vi "Set Dev Bounds.vi"(7 "error in (no error)":errorcluster, 8 "firmware revision":string(combo), 9 "dev bounds":T2={"dev bound upper cap (101)"=101.0, "dev bound upper loss (0.1)"=0.1, "dev bound lower cap (99)"=99.0, "dev bound lower loss (-0.1)"=-0.1}, 10 "VISA resource name":refnum<visa-resource-name>) -> (0 "error out":errorcluster, 2 "bridge error":T1, 3 "VISA resource name out":refnum<visa-resource-name>)   [LabVIEW 2019, in "Andeen-Hagerling 2700A.lvlib"]
doc: "Set the value of the value of the deviation mode bounds parameters.\n\nThis is the upper and lower bounds of the deviation capacitance\nand loss spans in pF and jpF respectively. The capacitance\nand loss bounds correspond directly to the analog output\nvoltage bounds for capacitance and loss respectively."
uses:
  Andeen-Hagerling 2700A.lvlib
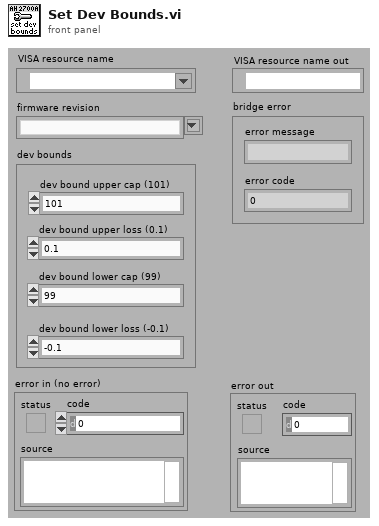
[diagram p1: front panel]
types:
  T1 = cluster{"error message":string, "error code":i32}
  T2 = cluster{"dev bound upper cap (101)":dbl, "dev bound upper loss (0.1)":dbl, "dev bound lower cap (99)":dbl, "dev bound lower loss (-0.1)":dbl}
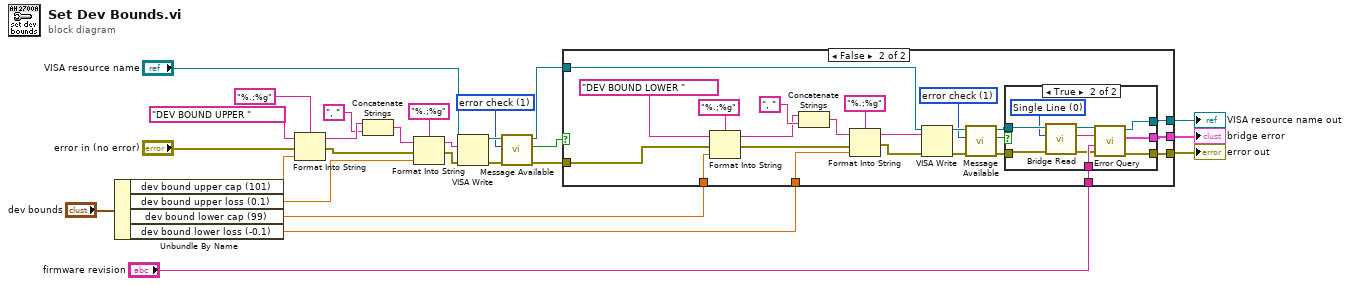
[diagram p0: block diagram]
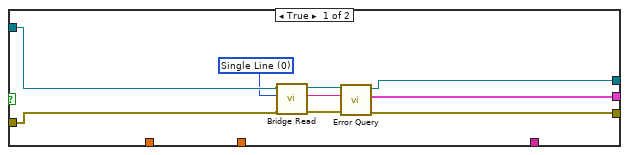
[diagram p2: hidden frame]
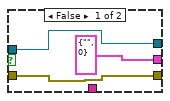
[diagram p3: hidden frame]
diagram:
  w1 = u16 1 items=["none", "error check", "multiline read", "infinite"] ("delay")
  n1 = Unbundle By Name("dev bounds") -> ("dev bound upper cap (101)"=w17:dbl, "dev bound upper loss (0.1)"=w16:dbl, "dev bound lower cap (99)"=w6:dbl, "dev bound lower loss (-0.1)"=w7:dbl)
  n2 = Format Into String(format string="%.;%g", initial string="DEV BOUND UPPER " ("command"), error in="error in (no error)", w17) -> (resulting string=w24:string, error out=w25:errorcluster)
  n3 = Concatenate Strings(w24, ", " ("command")) -> (w20:string)
  n4 = Format Into String(format string="%.;%g", initial string=w20, error in=w25, w16) -> (resulting string=w9:string, error out=w8:errorcluster)
  n5 = VISA Write(VISA resource name="VISA resource name", write buffer=w9, error in (no error)=w8) -> (VISA resource name out=w15:refnum<visa-resource-name>, error out=w14:errorcluster)  [unwired: 1 out]
  n6 = call "Message Available.vi"("error in (no error)"=w14, "delay"=w1, "VISA resource name"=w15) -> ("error out"=w12:errorcluster, "message available"=w11:bool, "VISA resource name out"=w13:refnum<visa-resource-name>)  [unwired: 6 in]
  n7 = case shown="False" w11 {
    tunnel: w6 -> [_ w44]
    tunnel: w7 -> [_ w43]
    tunnel: w13 -> [w29 w42]
    tunnel: "firmware revision" -> [_ w41]
    tunnel: [w35 w40] -> w4
    tunnel: [w34 w39] -> w3
    tunnel: [w33 w38] -> w2
    tunnel: w12 -> [w28 w37]
    frame True {
      w27 = u16 0 items=["Single Line", "Multi-Line"] ("Multiline")
      n8 = call "Bridge Read.vi"("error in (no error)"=w28, "multiline"=w27, "VISA resource name"=w29) -> ("error out"=w32:errorcluster, "read buffer"=w31:string, "VISA resource name out"=w30:refnum<visa-resource-name>)  [unwired: 6 in]
      n9 = call "Error Query.vi"("error in (no error)"=w32, "measurement line"=w31, "VISA resource name"=w30) -> ("error out"=w33:errorcluster, "bridge error"=w34:T1, "VISA resource name out"=w35:refnum<visa-resource-name>)  [unwired: 6 in]
    }
    frame False {
      w36 = u16 1 items=["none", "error check", "multiline read", "infinite"] ("delay")
      n10 = Format Into String(format string="%.;%g", initial string="DEV BOUND LOWER " ("command"), error in=w37, w44) -> (resulting string=w54:string, error out=w53:errorcluster)
      n11 = Concatenate Strings(w54, ", " ("command")) -> (w56:string)
      n12 = Format Into String(format string="%.;%g", initial string=w56, error in=w53, w43) -> (resulting string=w51:string, error out=w52:errorcluster)
      n13 = VISA Write(VISA resource name=w42, write buffer=w51, error in (no error)=w52) -> (VISA resource name out=w47:refnum<visa-resource-name>, error out=w46:errorcluster)  [unwired: 1 out]
      n14 = call "Message Available.vi"("error in (no error)"=w46, "delay"=w36, "VISA resource name"=w47) -> ("error out"=w48:errorcluster, "message available"=w50:bool, "VISA resource name out"=w49:refnum<visa-resource-name>)  [unwired: 6 in]
      n15 = case shown="True" w50 {
        tunnel: w49 -> [w60 w64]
        tunnel: w48 -> [w61 w63]
        tunnel: w41 -> [_ w71]
        tunnel: [w61 w70] -> w38
        tunnel: [w60 w69] -> w40
        tunnel: [T1 {"error message"="", "error code"=0} ("bridge error") w68] -> w39
        frame False {
        }
        frame True {
          w62 = u16 0 items=["Single Line", "Multi-Line"] ("Multiline")
          n16 = call "Bridge Read.vi"("error in (no error)"=w63, "multiline"=w62, "VISA resource name"=w64) -> ("error out"=w67:errorcluster, "read buffer"=w66:string, "VISA resource name out"=w65:refnum<visa-resource-name>)  [unwired: 6 in]
          n17 = call "Error Query.vi"("error in (no error)"=w67, "firmware revision"=w71, "measurement line"=w66, "VISA resource name"=w65) -> ("error out"=w70:errorcluster, "bridge error"=w68:T1, "VISA resource name out"=w69:refnum<visa-resource-name>)  [unwired: 5 in]
        }
      }
    }
  }
  "VISA resource name out" <- w4
  "error out" <- w2
  "bridge error" <- w3
